vi "Move Toward Nearest Wall.vi"(9 "Column":i32, 10 "Row":i32, 11 "private data in":T2) -> (0 "nearest wall":T1, 1 "front line?":bool, 2 "goal angle (deg)":dbl, 3 "private data out":T2)   [LabVIEW 2020, in "Great Wall.lvclass"]
uses:
  Great Wall.lvclass
  Private Data.ctl
  Wall State.ctl
  Wall State Enum.ctl
  Type Defs/Direction Enum.ctl
  DS Square Library/DS Square.lvlib
  Type Defs/SB Type Defs.lvlib
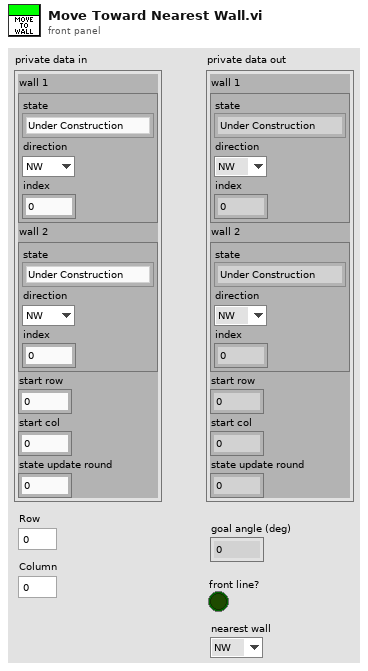
[diagram p1: front panel]
types:
  T1 = typedef "SB Type Defs.lvlib/Direction Enum.ctl" = enum16{"NW", "N", "NE", "E", "SE", "S", "SW", "W"}
  T2 = typedef "Great Wall.lvclass/Private Data.ctl" = cluster{"wall 1":T3, "wall 2":T3, "start row":i32, "start col":i32, "state update round":i32}
  T3 = typedef "Great Wall.lvclass/Wall State.ctl" = cluster{"state":T4, "direction":T1, "index":i32}
  T4 = typedef "Great Wall.lvclass/Wall State Enum.ctl" = enum16{"Under Construction", "Hold", "Advance 1", "Advance 2", "Retreat"}
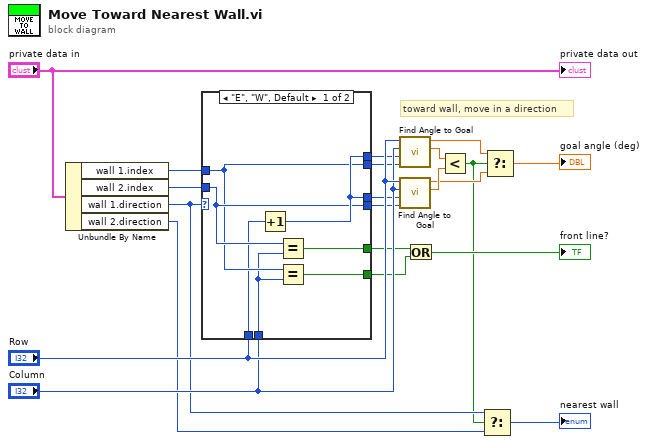
[diagram p0: block diagram]
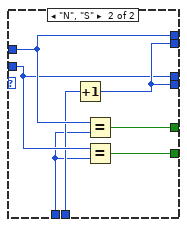
[diagram p2: hidden frame]
diagram:
  # "toward wall, move in a direction"
  n1 = Unbundle By Name("private data in") -> ("wall 1.index"=w20:i32, "wall 2.index"=w21:i32, "wall 1.direction"=w3:T1, "wall 2.direction"=w4:T1)
  n2 = case shown="\"E\", \"W\", Default" w3 {
    tunnel: "Row" -> [w25 w29]
    tunnel: "Column" -> [w22 w30]
    tunnel: w21 -> [w27 w31]
    tunnel: w20 -> [w26 w32]
    tunnel: [w28 w32] -> w17
    tunnel: [w28 w31] -> w16
    tunnel: [w27 w35] -> w15
    tunnel: [w26 w35] -> w14
    tunnel: [w24 w34] -> w7
    tunnel: [w23 w33] -> w5
    frame "E", "W", Default {
      n3 = Increment(x=w25) -> (x+1=w28:i32)
      n4 = Equal?(x=w27, y=w22) -> (x = y?=w24:bool)
      n5 = Equal?(x=w26, y=w22) -> (x = y?=w23:bool)
    }
    frame "N", "S" {
      n6 = Increment(x=w30) -> (x+1=w35:i32)
      n7 = Equal?(x=w32, y=w29) -> (x = y?=w34:bool)
      n8 = Equal?(x=w31, y=w29) -> (x = y?=w33:bool)
    }
  }
  n9 = call "Find Angle to Goal.vi"("Goal Column"=w14, "Goal Row"=w17, "Column"="Column", "Row"="Row") -> ("distance"=w13:dbl, "angle (deg)"=w11:dbl)  [unwired: 4 in, 2 out]
  n10 = call "Find Angle to Goal.vi"("Goal Column"=w15, "Goal Row"=w16, "Column"="Column", "Row"="Row") -> ("distance"=w12:dbl, "angle (deg)"=w10:dbl)  [unwired: 4 in, 2 out]
  n11 = Or(x=w7, y=w5) -> (x .or. y?=→"front line?":bool)
  n12 = Less?(x=w13, y=w12) -> (x < y?=w1:bool)
  n13 = Select(t=w3, s=w1, f=w4) -> (s? t:f=→"nearest wall":T1)
  n14 = Select(t=w11, s=w1, f=w10) -> (s? t:f=→"goal angle (deg)":dbl)
  "private data out" <- "private data in"
